vi "connect.vi"(8 "error in (no error)":errorcluster, 10 "Serial Port":refnum<visa-resource-name>, 11 "MotorController in":refnum<class "MotorController.lvclass">) -> (0 "error out":errorcluster, 3 "MotorController out":refnum<class "MotorController.lvclass">)   [LabVIEW 2019, in "MotorController.lvclass"]
uses:
  MotorController.lvclass
  MotorController.lvclass/MotorController.ctl
  <vilib>/Instr/_visa.llb/VISA Configure Serial Port (Instr).vi
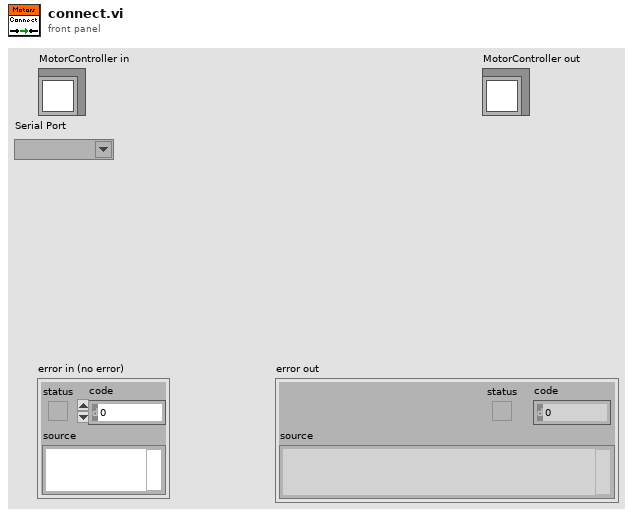
[diagram p1: front panel]
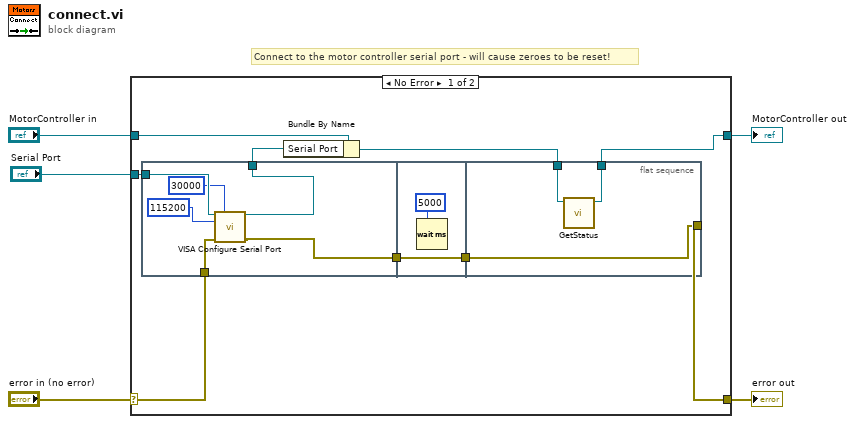
[diagram p0: block diagram]
diagram:
  # "Connect to the motor controller serial port - will cause zeroes to be reset!"
  n1 = case shown="No Error" "error in (no error)" {
    selector: "error in (no error)" -> [w13 w27]
    tunnel: [w8 w27] -> w4
    tunnel: [w6 w26] -> w2
    tunnel: "MotorController in" -> [w12 w26]
    tunnel: "Serial Port" -> [w14 _]
    frame No Error {
      n2 = flat-sequence {
        tunnel: w14 -> [w19]
        tunnel: w13 -> [w18]
        tunnel: [w17] -> w11
        tunnel: [w16] -> w9
        tunnel: [w21] -> w10
        tunnel: w9 -> [w21]
        tunnel: w7 -> [w25]
        tunnel: w10 -> [w23]
        tunnel: [w23] -> w8
        tunnel: [w24] -> w6
        frame #0 {
          n3 = call-poly "VISA Configure Serial Port"("VISA resource name"=w19, "timeout (10sec)"=u32 30000, "baud rate (9600)"=u32 115200, "error in (no error)"=w18) -> ("VISA resource name out"=w17:refnum<visa-resource-name>, "error out"=w16:errorcluster)  [unwired: 10 in]
        }
        frame #1 {
          n4 = Wait (ms)(milliseconds to wait=u32 5000) -> ()  [unwired: 1 out]
        }
        frame #2 {
          n5 = call "GetStatus.vi"("MotorController in"=w25) -> ("MotorController out"=w24:refnum<class "MotorController.lvclass">)  [unwired: 8 in, 2 out]
        }
      }
      n6 = Bundle By Name(cluster=w12, "Serial Port"=w11) -> (w7:refnum<class "MotorController.lvclass">)
    }
    frame Error {
    }
  }
  "error out" <- w4
  "MotorController out" <- w2
